vi "Dynamic Block Lock 1k.vi"(9 "Dynamic Block Lock Page Section 1K":T1, 11 "PN532 COM Port":refnum<visa-resource-name>) -> (0 "Error out":errorcluster, 2 "Succeeded":bool, 3 "PN532 COM Port Out":refnum<visa-resource-name>)   [LabVIEW 2012, in "NFC Driver.lvlib"]
uses:
  NFC Driver.lvlib
  Typedef/Dynamic Block Lock Page Section 1K.ctl
panel:
  out "result string":string
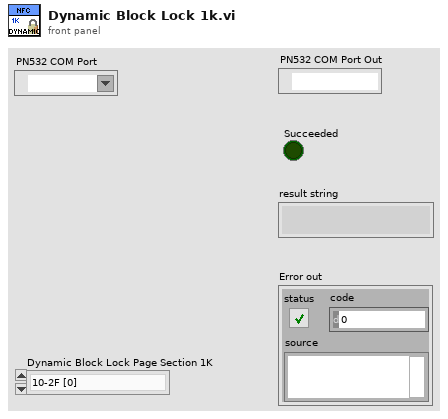
[diagram p1: front panel]
types:
  T1 = typedef "NFC Driver.lvlib/Dynamic Block Lock Page Section 1K.ctl" = enum16{"10-2F [0]", "30-4F [1]", "50-6F [2]", "70-8F [3]", "90-AF [4]", "B0-CF [5]", "D0-E1 [6]"}
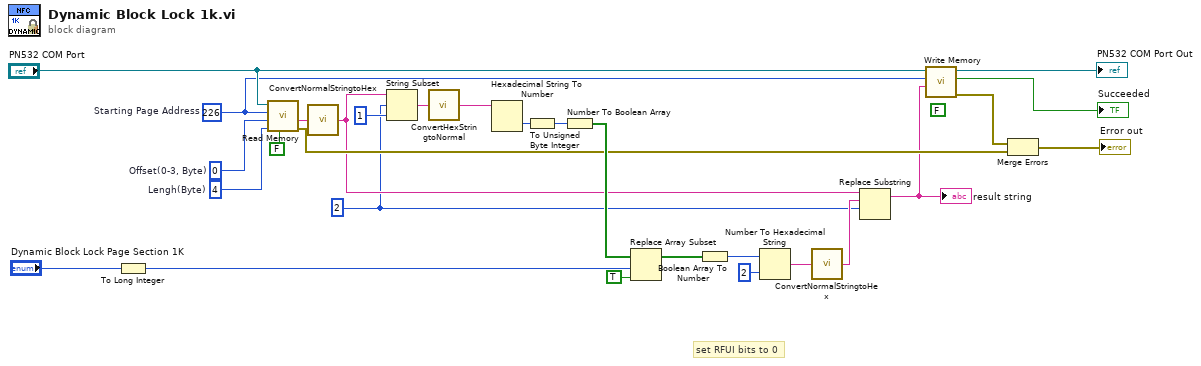
[diagram p0: block diagram]
diagram:
  w4 = 2 ("offset (0)")
  w5 = 0  # Offset(0-3, Byte)
  (unwired) FALSE ("Data in ASCII")
  w25 = 4  # Lengh(Byte)
  w11 = 226  # Starting Page Address
  # "set RFUI bits to 0"
  n1 = To Long Integer(number="Dynamic Block Lock Page Section 1K") -> (32bit integer=w8:i32)
  n2 = call "Read Memory.vi"("Reverse Output[F]"=FALSE, "length (Byte, max. 16)"=w25, "offset (Byte, max. 16)"=w5, "Page Address"=w11, "PN532 COM Port"="PN532 COM Port") -> ("error out"=w19:errorcluster, "Selected substring (HEX)"=w1:string)  [unwired: 2 in, 3 out]
  n3 = call "ConvertNormalStringtoHex.vi"("Normal String"=w1) -> ("Hex String"=w10:string)
  n4 = String Subset(string=w10, offset (0)=w4, length (rest)=1 ("length (rest)")) -> (substring=w13:string)
  n5 = call "ConvertHexStringtoNormal.vi"("Hex String"=w13) -> ("Normal String"=w12:string)
  n6 = Hexadecimal String To Number(string=w12) -> (number=w24:u32)  [unwired: 2 in, 1 out]
  n7 = To Unsigned Byte Integer(number=w24) -> (unsigned 8bit integer=w15:u8)
  n8 = Number To Boolean Array(number=w15) -> (Boolean array=w23:bool[])
  n9 = Replace Array Subset(array=w23, new element=TRUE ("new element/subarray"), index=w8) -> (w18:bool[])
  n10 = Boolean Array To Number(Boolean array=w18) -> (number=w22:u32)
  n11 = Number To Hexadecimal String(1:i16 2 ("width (-)"), 2:w22) -> (0:w9:string)
  n12 = call "ConvertNormalStringtoHex.vi"("Normal String"=w9) -> ("Hex String"=w6:string)
  n13 = Replace Substring(3:w4, 4:w6, 5:w10) -> (1:w7:string)  [unwired: 1 in, 1 out]
  "result string" <- w7
  n14 = call "Write Memory.vi"("Data to write (HEX, max 16 bytes)"=w7, "Page Address"=w11, "PN532 COM Port"="PN532 COM Port") -> ("Error Out"=w20:errorcluster, "Succesful?"=→"Succeeded":bool, "PN532 COM Port Out"=→"PN532 COM Port Out":refnum<visa-resource-name>)  [unwired: 6 in]
  n15 = Merge Errors(w20, w19) -> (→"Error out":errorcluster)
